vi "Receive Value Change Msg.vi"(8 "error in (no error)":errorcluster, 10 "ValueChangeMsg":refnum<class "ValueChangeMsg.lvclass">, 11 "TopLevelApplication In":refnum<class "ConcreteViewModel.lvclass">) -> (0 "error out":errorcluster, 3 "TopLevelApplication Out":refnum<class "ConcreteViewModel.lvclass">)   [LabVIEW 2015, in "TopLevelApplication.lvlib" / "ConcreteViewModel.lvclass"]
doc: "<License>\nCopyright © 2017 Composed Systems, LLC | All rights reserved\nwww.composed.io\n\nAuthor: Ethan Stern <ethan.stern@composed.io>\n\nThis software is provided \"AS IS\" WITHOUT WARRANTIES, either express or implied, AND IS FOR EDUCATIONAL PURPOSES ONLY.\n</License>"
uses:
  ConcreteViewModel.lvclass
  Framework/AutoRegistration/ActorAutoRegistration Messages/ValueChangeMsg/ValueChangeMsg.lvclass
  <vilib>/Utility/Data Type/NI_Data Type.lvlib
  Dialog Box Implementations/OneButtonDialogBox/OneButtonDialogBox.lvclass
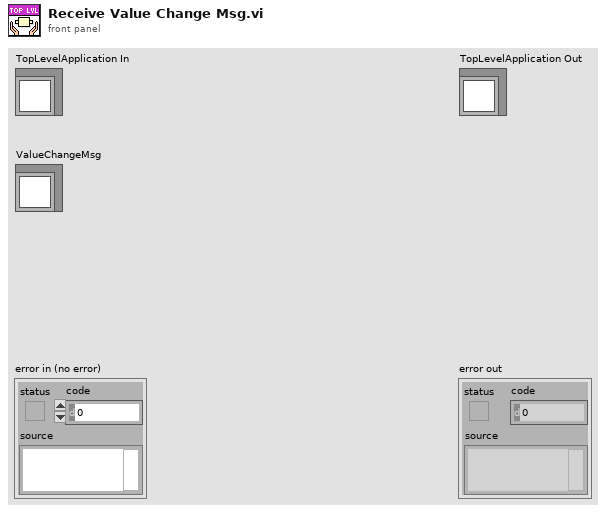
[diagram p1: front panel]
types:
  T1 = typedef "NI_Data Type.lvlib/Data Type.ctl" = enum8{"Invalid Type", "Void", "I8", "I16", "I32", "I64", "U8", "U16", "U32", "U64", "Single Float", "Double Float", "Extended Float", "Single Complex", "Double Complex", "Extended Complex", "Enum U8", "Enum U16", "Enum U32", "Enum U64", "Single Float With Unit", "Double Float With Unit", "Extended Float With Unit", "Single Complex with Unit", "Double Complex with Unit", "Extended Complex with Unit", "Boolean", "String", "Path", "Picture", "Tag", "Array", "Cluster", "Variant", "LV Variant", "Waveform", "Timestamp", "Digital Waveform", "Digital Data", "ExpressData", "Refnum", "External Data", "VI", "Poly VI", "LabVIEW Class Instance", "Fixed Point"}
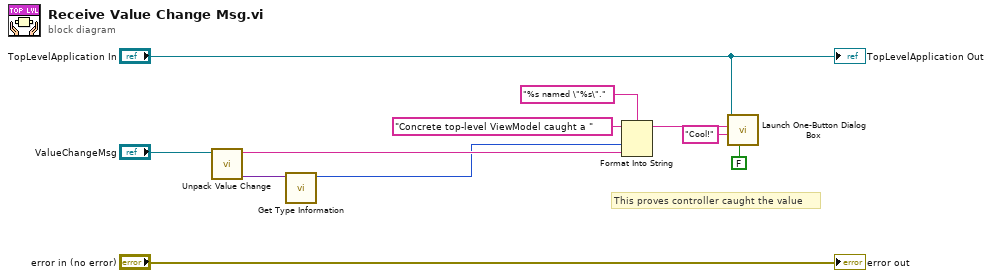
[diagram p0: block diagram]
diagram:
  # "This proves controller caught the value"
  n1 = call-dynamic "Unpack Value Change.vi"("ValueChangeMsg In"="ValueChangeMsg") -> ("New Value"=w3:variant, "Name"=w7:string)  [unwired: 7 in, 2 out]
  n2 = call <vilib>:"Get Type Information.vi"("Variant"=w3) -> ("Type"=w2:T1)  [unwired: 6 in, 4 out]
  n3 = Format Into String(format string="%s named \"%s\".", initial string="Concrete top-level ViewModel caught a ", w2, w7) -> (resulting string=w5:string)  [unwired: 1 in, 1 out]
  n4 = call "Launch One-Button Dialog Box.vi"("Modal? (T)"=FALSE, "Button Text (OK)"="Cool!", "Message Text"=w5, "Dialog Launcher"="TopLevelApplication In") -> ()  [unwired: 7 in, 1 out]
  "error out" <- "error in (no error)"
  "TopLevelApplication Out" <- "TopLevelApplication In"
